vi "KE622x -- Set Op Event Enable Reg State.vi"(0 "VISA Resource In":refnum<visa-resource-name>, 1 "Error Query (T)?":bool=TRUE, 7 "KE622x Op Event Enable Reg":T1, 11 "error in (no error)":errorcluster) -> (4 "VISA Resource Out (dupl)":refnum<visa-resource-name>, 15 "error out":errorcluster)   [LabVIEW 2019, in "Keithley 622x.lvlib"]
doc: "Sets the bits in the 'Operation Event Enable' register of the Status Model. Note that only the used (named) bits are settable -- all other bits default to zero."
uses:
  Keithley 622x.lvlib
  Typedefs/KE622x -- Op Event Enable Reg State.ctl
panel:
  out "Reg Num (dec)":u16 format="%0d"
  out "Reg Num (binary)":u16 format="%016b"
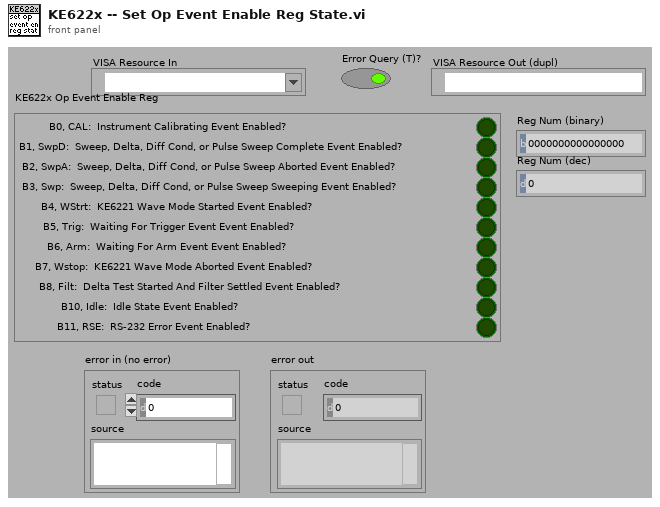
[diagram p1: front panel]
types:
  T1 = typedef "Keithley 622x.lvlib/KE622x -- Op Event Enable Reg State.ctl" = cluster{"B0, CAL:  Instrument Calibrating Event Enabled?":bool, "B1, SwpD:  Sweep, Delta, Diff Cond, or Pulse Sweep Complete Event Enabled?":bool, "B2, SwpA:  Sweep, Delta, Diff Cond, or Pulse Sweep Aborted Event Enabled?":bool, "B3, Swp:  Sweep, Delta, Diff Cond, or Pulse Sweep Sweeping Event Enabled?":bool, "B4, WStrt:  KE6221 Wave Mode Started Event Enabled?":bool, "B5, Trig:  Waiting For Trigger Event Event Enabled?":bool, "B6, Arm:  Waiting For Arm Event Event Enabled?":bool, "B7, Wstop:  KE6221 Wave Mode Aborted Event Enabled?":bool, "B8, Filt:  Delta Test Started And Filter Settled Event Enabled?":bool, "B10, Idle:  Idle State Event Enabled?":bool, "B11, RSE:  RS-232 Error Event Enabled?":bool}
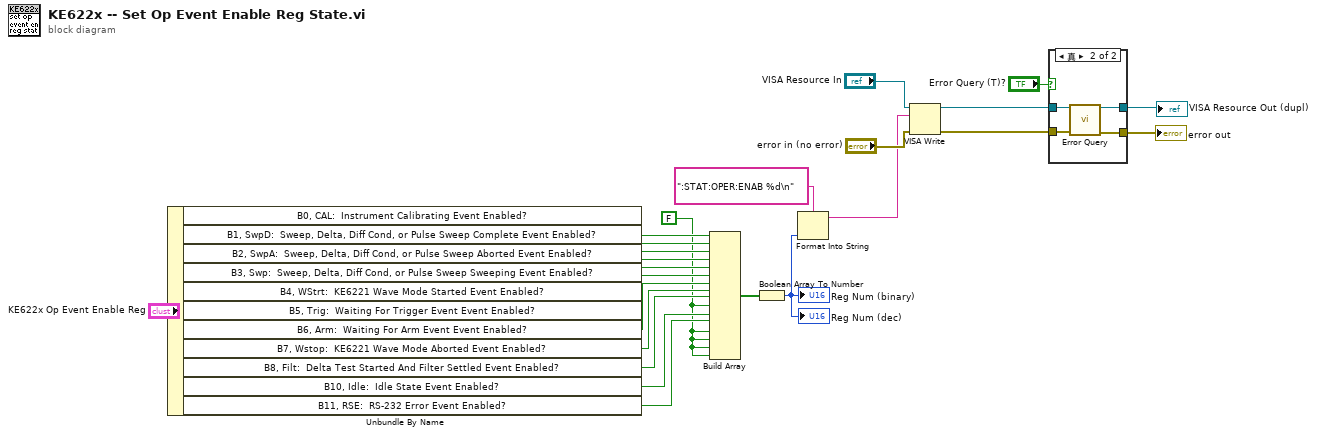
[diagram p0: block diagram]
diagram:
  w1 = FALSE
  n1 = Unbundle By Name("KE622x Op Event Enable Reg") -> ("B0, CAL:  Instrument Calibrating Event Enabled?"=w12:bool, "B1, SwpD:  Sweep, Delta, Diff Cond, or Pulse Sweep Complete Event Enabled?"=w11:bool, "B2, SwpA:  Sweep, Delta, Diff Cond, or Pulse Sweep Aborted Event Enabled?"=w10:bool, "B3, Swp:  Sweep, Delta, Diff Cond, or Pulse Sweep Sweeping Event Enabled?"=w9:bool, "B4, WStrt:  KE6221 Wave Mode Started Event Enabled?"=w8:bool, "B5, Trig:  Waiting For Trigger Event Event Enabled?"=w7:bool, "B6, Arm:  Waiting For Arm Event Event Enabled?"=w6:bool, "B7, Wstop:  KE6221 Wave Mode Aborted Event Enabled?"=w5:bool, "B8, Filt:  Delta Test Started And Filter Settled Event Enabled?"=w4:bool, "B10, Idle:  Idle State Event Enabled?"=w3:bool, "B11, RSE:  RS-232 Error Event Enabled?"=w2:bool)
  n2 = Build Array(w12, w11, w10, w9, w8, w7, w6, w5, w4, w1, w3, w2, w1, w1, w1, w1) -> (w24:bool[])
  n3 = Boolean Array To Number(Boolean array=w24) -> (number=w21:u32)
  "Reg Num (binary)" <- w21
  "Reg Num (dec)" <- w21
  n4 = Format Into String(format string=":STAT:OPER:ENAB %d\n" ("write buffer"), w21) -> (resulting string=w19:string)  [unwired: 2 in, 1 out]
  n5 = VISA Write(VISA resource name="VISA Resource In", write buffer=w19, error in (no error)="error in (no error)") -> (VISA resource name out=w17:refnum<visa-resource-name>, error out=w18:errorcluster)  [unwired: 1 out]
  n6 = case shown="真" "Error Query (T)?" {
    tunnel: w18 -> [w25 w30]
    tunnel: w17 -> [w26 w29]
    tunnel: [w25 w28] -> w16
    tunnel: [w26 w27] -> w15
    frame False {
    }
    frame True {
      n7 = call "Error Query.vi"("VISA Resource In"=w29, "error in (no error)"=w30) -> ("VISA Resource Out (dupl)"=w27:refnum<visa-resource-name>, "error out"=w28:errorcluster)  [unwired: 10 in, 2 out]
    }
  }
  "VISA Resource Out (dupl)" <- w15
  "error out" <- w16
